vi "checkTimeOut.vi"(8 "error in (no error)":errorcluster, 10 "Time":u32, 11 "ParameterConf in":refnum<class "ParameterConf.lvclass">) -> (0 "error out":errorcluster, 2 "timeout":bool, 3 "ParameterConf out":refnum<class "ParameterConf.lvclass">)   [LabVIEW 2017, in "LibraryGcode.lvlib" / "ParameterConf.lvclass"]
uses:
  ParameterConf.lvclass
  ParameterConf.lvclass/ParameterConf.ctl
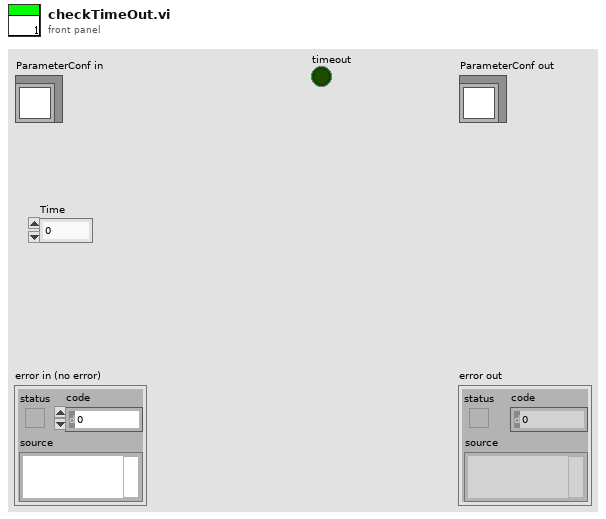
[diagram p1: front panel]
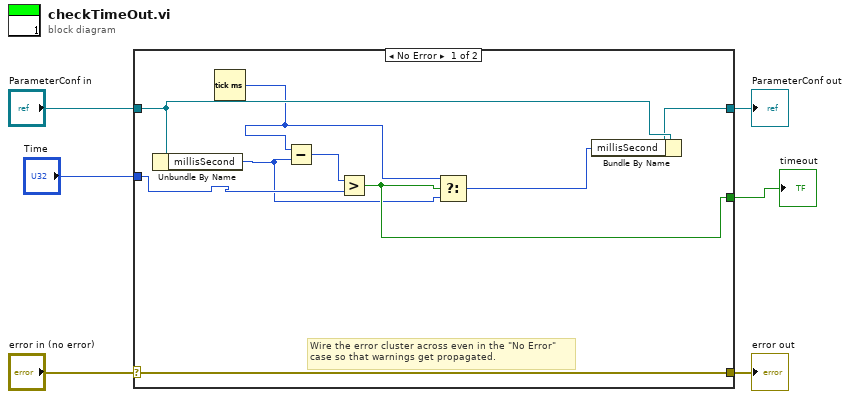
[diagram p0: block diagram]
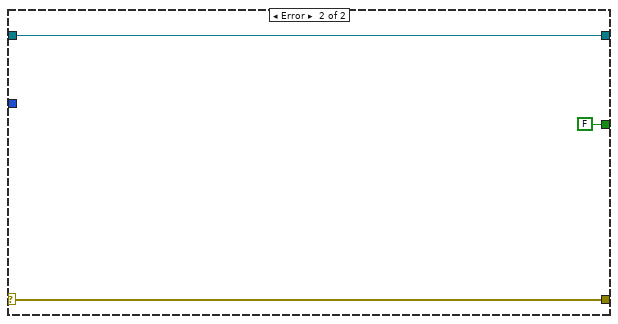
[diagram p2: hidden frame]
diagram:
  n1 = case shown="No Error" "error in (no error)" {
    selector: "error in (no error)" -> [w15 w18]
    tunnel: [w15 w18] -> w5
    tunnel: [w12 w17] -> w3
    tunnel: "ParameterConf in" -> [w13 w17]
    tunnel: "Time" -> [w8 _]
    tunnel: [w11 FALSE] -> w1
    frame No Error {
      # "Wire the error cluster across even in the \"No Error\"\ncase so that warnings get propagated."
      n2 = Unbundle By Name(w13) -> ("millisSecond"=w7:u32)
      n3 = Tick Count (ms)() -> (millisecond timer value=w9:u32)
      n4 = Subtract(x=w9, y=w7) -> (x-y=w14:u32)
      n5 = Greater?(x=w14, y=w8) -> (0:w11:bool)
      n6 = Select(t=w9, s=w11, f=w7) -> (s? t:f=w10:u32)
      n7 = Bundle By Name(cluster=w13, "millisSecond"=w10) -> (w12:refnum<class "ParameterConf.lvclass">)
    }
    frame Error {
    }
  }
  "error out" <- w5
  "ParameterConf out" <- w3
  "timeout" <- w1
